vi "Move Controller-v2.vi"(5 "Move Control":T1={"Down"=FALSE, "Up"=FALSE, "Right"=FALSE, "Left"=FALSE, "APulses X"=100, "APulses Y"=100, "Stop"=FALSE}, 6 "Reverse":cluster{"Reverse X":bool, "Reverse Y":bool}) -> (0 "Go":bool, 1 "APulses":u16, 2 "Direction":bool, 3 "Axis (X=1,Y=2,Z=3)":u16, 4 "Stop":bool)   [LabVIEW 2013]
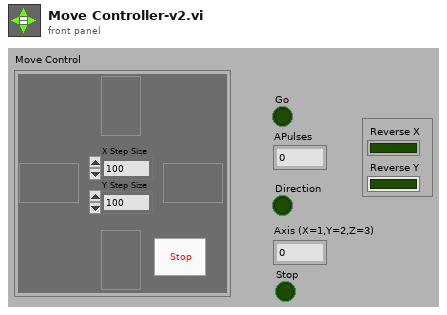
[diagram p1: front panel]
types:
  T1 = cluster{"Down":bool, "Up":bool, "Right":bool, "Left":bool, "APulses X":u16, "APulses Y":u16, "Stop":bool}
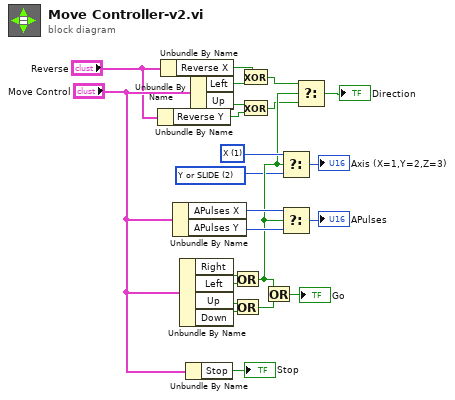
[diagram p0: block diagram]
diagram:
  w1 = u16 2 items=["X"=1, "Y or SLIDE"=2, "Z"=3] ("AXIS")
  w21 = u16 1 items=["X"=1, "Y or SLIDE"=2, "Z"=3] ("AXIS")
  n1 = Unbundle By Name("Reverse") -> ("Reverse Y"=w2:bool)
  n2 = Unbundle By Name("Reverse") -> ("Reverse X"=w4:bool)
  n3 = Unbundle By Name("Move Control") -> ("APulses X"=w12:u16, "APulses Y"=w11:u16)
  n4 = Unbundle By Name("Move Control") -> ("Right"=w15:bool, "Left"=w16:bool, "Up"=w18:bool, "Down"=w17:bool)
  n5 = Unbundle By Name("Move Control") -> ("Stop"=→"Stop":bool)
  n6 = Unbundle By Name("Move Control") -> ("Left"=w20:bool, "Up"=w19:bool)
  n7 = Or(x=w15, y=w16) -> (x .or. y?=w8:bool)
  n8 = Or(x=w18, y=w17) -> (x .or. y?=w14:bool)
  n9 = Exclusive Or(1:w20, 2:w4) -> (0:w9:bool)
  n10 = Exclusive Or(1:w2, 2:w19) -> (0:w7:bool)
  n11 = Or(x=w8, y=w14) -> (x .or. y?=→"Go":bool)
  n12 = Select(t=w21, s=w8, f=w1) -> (s? t:f=→"Axis (X=1,Y=2,Z=3)":u16)
  n13 = Select(t=w12, s=w8, f=w11) -> (s? t:f=→"APulses":u16)
  n14 = Select(t=w9, s=w8, f=w7) -> (s? t:f=→"Direction":bool)
